vi "TEST FGV User Event Reference Manager.vi"(8 "error in (no error)":errorcluster) -> (0 "error out":errorcluster)   [LabVIEW 2011]
doc: "This is the solution for one of a two VI test process for the FGV User Event Reference.vi. This VI allows the operator to create an undertermined number of User Events and fire those User Events.\n\nAAL 9/09"
uses:
  Type Defs/TYPE FGV User Event Method.ctl
  Shared/QDMH Poly VIs/QDMH POLY Enqueue String.vi
panel:
  in  "Queue Name":string
  in  "Fire User Event":bool
  in  "User Event Ref to Act Upon":u16(ring)
  in  "Delete User Event":bool
  in  "Add User Event":bool
  out "Message Display":string
  in  "Cancel":bool
  in  "OK":bool
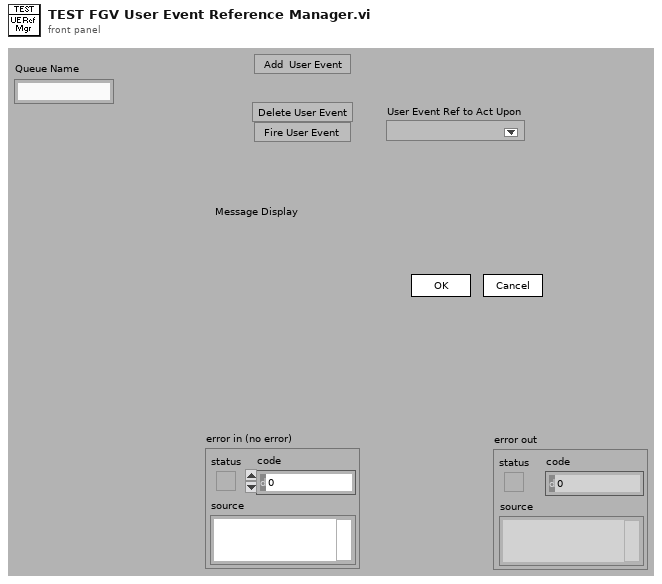
[diagram p1: front panel]
types:
  T1 = cluster{"Operator Name":string, "Current VI's Path":path, "# User Event  Refs":i32, "User Event #":i32, "User Event Names":string[], "User Event to Act Upon":i32}
  T2 = typedef "TYPE FGV User Event Method.ctl" = enum16{"Add User Event Ref", "Get User Event Ref", "Delete User Event Ref", "Get All User Event Refs", "Delete All User Event Refs"}
  T3 = typedef "TYPE FGV User Event Ref.ctl" = refnum<user-event>
  T4 = cluster{"User Event Name":string, "Variant":variant}
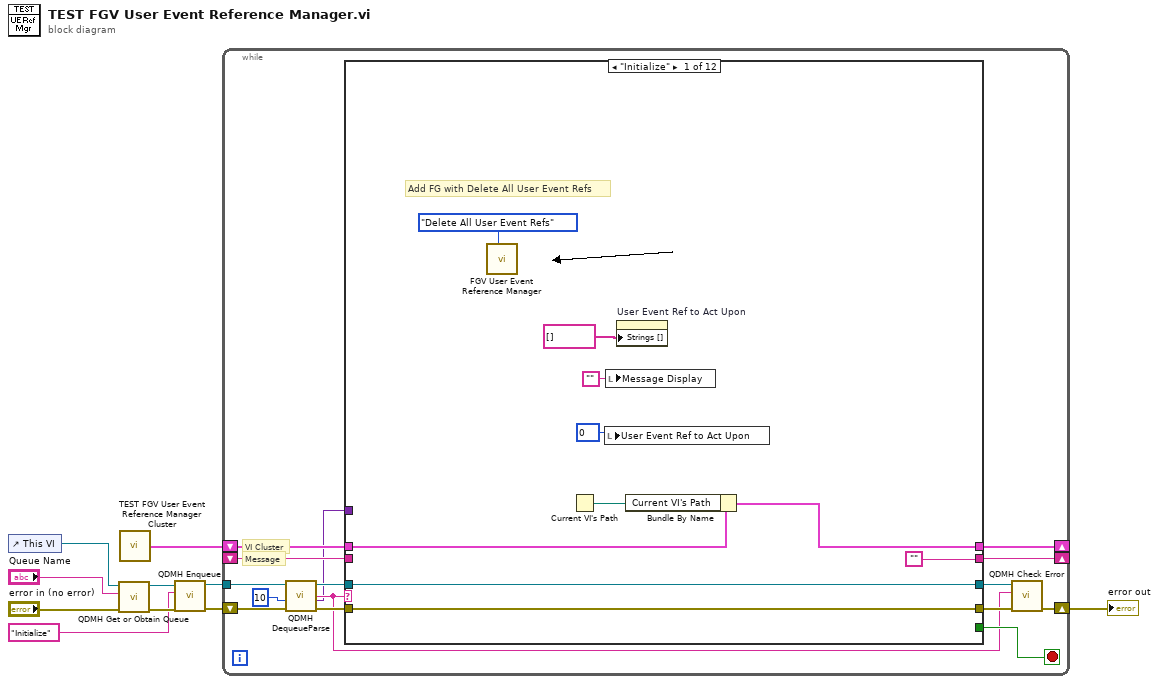
[diagram p0: block diagram]
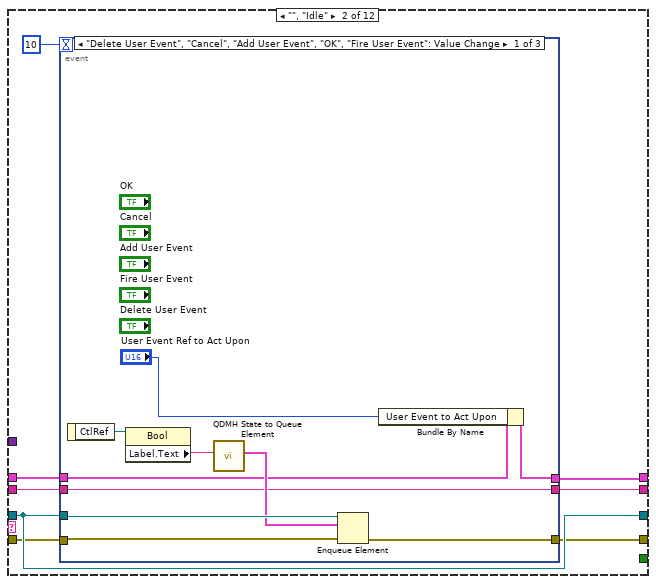
[diagram p2: hidden frame]
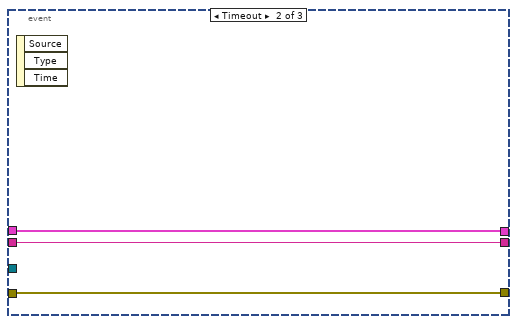
[diagram p3: hidden frame]
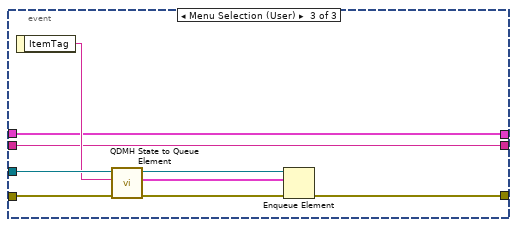
[diagram p4: hidden frame]
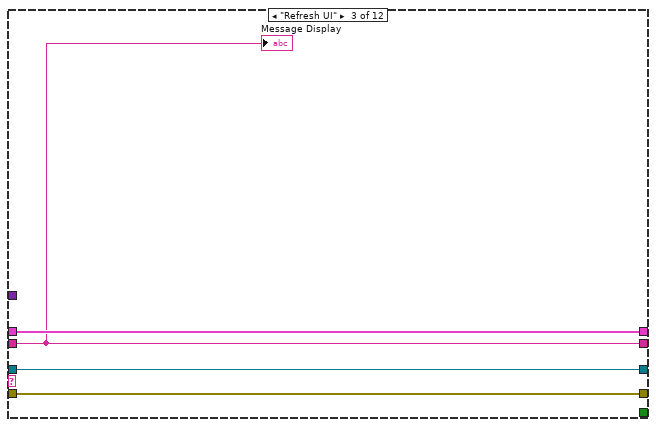
[diagram p5: hidden frame]
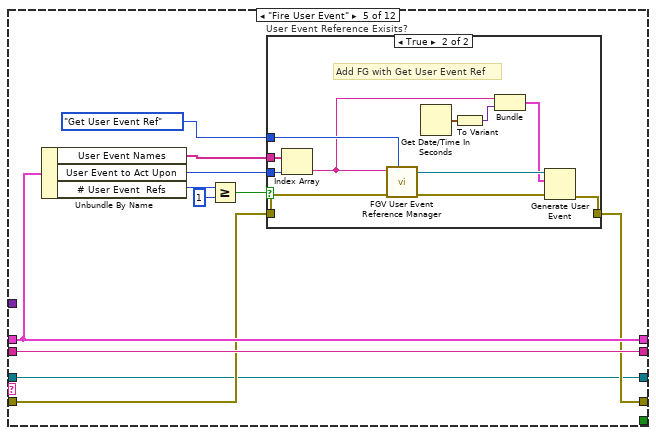
[diagram p7: hidden frame]
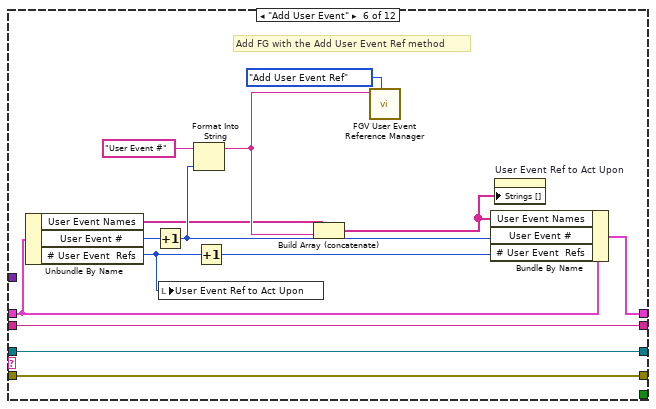
[diagram p9: hidden frame]
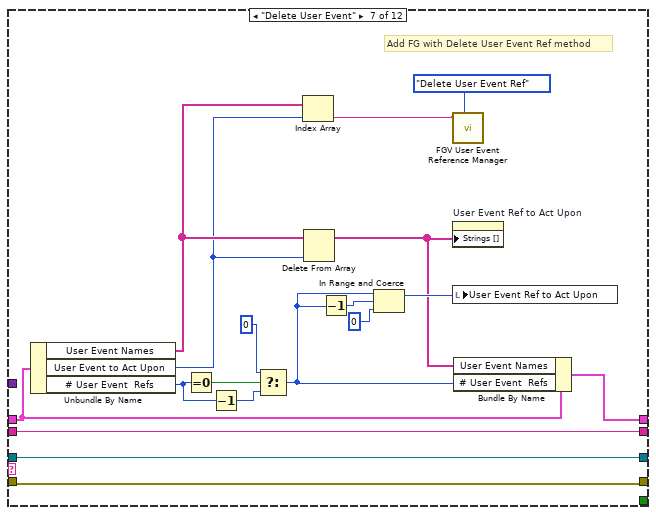
[diagram p10: hidden frame]
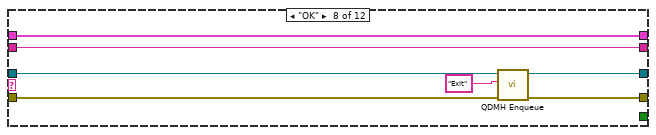
[diagram p11: hidden frame]
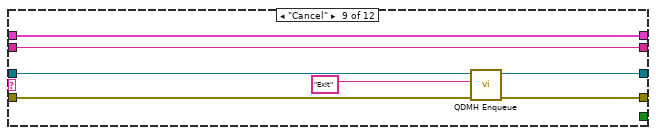
[diagram p12: hidden frame]
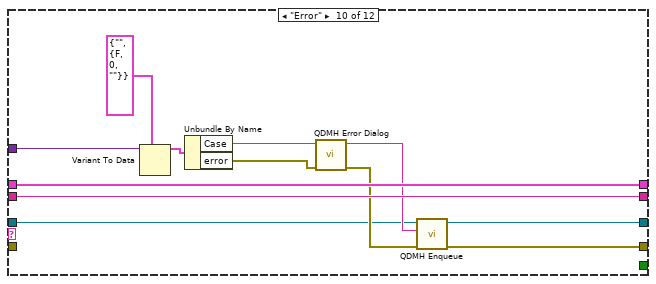
[diagram p13: hidden frame]
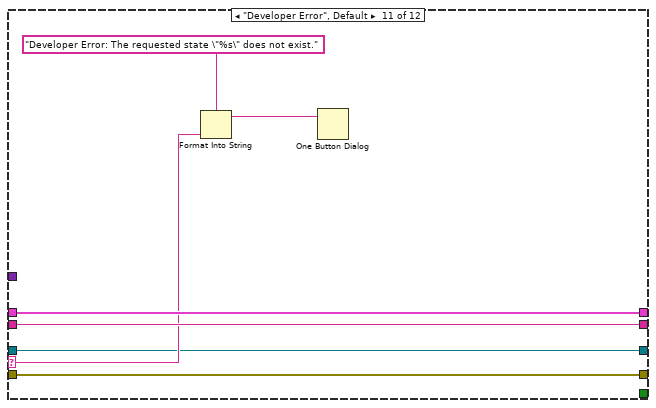
[diagram p14: hidden frame]
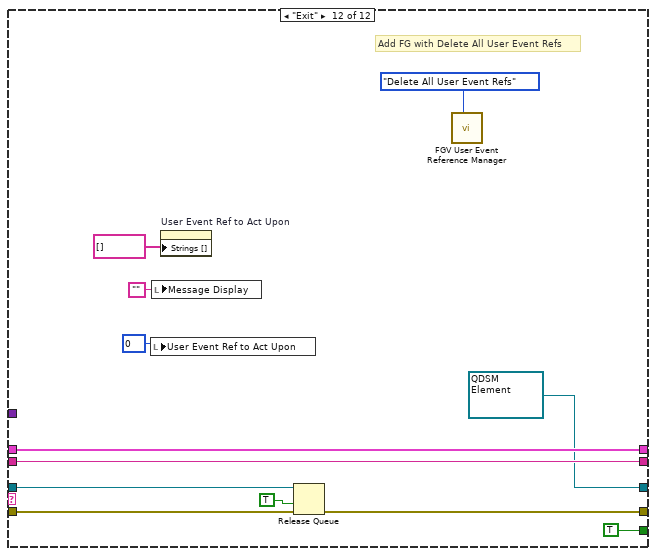
[diagram p15: hidden frame]
diagram:
  n1 = control-ref of="This VI"() -> (w2:refnum<vi>)
  n2 = call "QDMH Get or Obtain Queue.vi"("error in (no error)"="error in (no error)", "Queue Name"="Queue Name", "VI Refnum"=w2) -> ("error out"=w6:errorcluster, "queue out"=w9:refnum<queue>)  [unwired: 7 out]
  n3 = call "TEST FGV User Event Reference Manager Cluster.vi"() -> ("Cluster"=w8:T1)
  n4 = call-poly "QDMH Enqueue.vi"("error in (no error)"=w6, "State"="Initialize" ("element"), "queue"=w9) -> ("error out"=w7:errorcluster, "queue out"=w10:refnum<queue>)  [unwired: 7 out]
  n5 = while {
    tunnel: w10 -> [w21]
    shift-left: w8 -> [w22]
    shift-right: [w23] -> _
    shift-left: _ -> [w24]
    shift-right: [w15] -> _
    shift-right: [w13] -> w4
    shift-left: w7 -> [w17]
    stop <- w25 stop-if-true
    # "VI Cluster"
    # "Message"
    n6 = call "QDMH DequeueParse.vi"("error in (no error)"=w17, "Timeout"=10 ("ms timeout (-1)"), "queue"=w21) -> ("error out"=w18:errorcluster, "Variant Data"=w11:variant, "State"=w12:string, "queue out"=w19:refnum<queue>)  [unwired: 5 out]
    n7 = case shown="\"Initialize\"" w12 {
      selector: w12 -> [_ _ _ _ _ _ _ _ _ _ w156 _]
      tunnel: w19 -> [w26 w43 w64 w68 w72 w95 w109 w133 w140 w142 w153 w161]
      tunnel: [_ _ _ _ _ _ _ _ _ _ _ TRUE] -> w25
      tunnel: ["" w37 w66 w71 w82 w108 w126 w132 w139 w152 w159 w170] -> w15
      tunnel: w24 -> [_ w38 w66 w71 w82 w108 w126 w132 w139 w152 w159 w170]
      tunnel: [w33 w36 w67 w70 w81 w105 w124 w131 w138 w151 w158 w169] -> w23
      tunnel: w22 -> [w34 w39 w67 w70 w81 w106 w125 w131 w138 w151 w158 w169]
      tunnel: w18 -> [w35 w42 w65 w69 w77 w96 w111 w130 w137 _ w155 w167]
      tunnel: [w35 w41 w65 w69 w76 w96 w111 w129 w136 w143 w155 w166] -> w16
      tunnel: [w26 w43 w64 w68 w72 w95 w109 w127 w134 w144 w153 refnum<queue> refnum ("queue out")] -> w14
      tunnel: w11 -> [_ _ _ _ _ _ _ _ _ w141 _ _]
      frame "Initialize" {
        w28 = u16 0 items=[""] ("Queue to Delete")
        # "Add FG with Delete All User Event Refs"
        n8 = call "FGV User Event Reference Manager.vi"("Method (Get User Event Ref)"=TYPE_FGV_User_Event_Method."Delete All User Event Refs") -> ()  [unwired: 2 in, 9 out]
        n9 = Current VI's Path() -> (path=w32:path)
        n10 = local write "User Event Ref to Act Upon"(w28) -> ()
        n11 = local write "Message Display"("") -> ()
        n12 = property on="User Event Ref to Act Upon" class="Ring (strict)"("Strings []"=string[] []) -> ()  [unwired: 2 in, 2 out]
        n13 = Bundle By Name(cluster=w34, "Current VI's Path"=w32) -> (w33:T1)
      }
      frame "", "Idle" {
        n14 = event shown="[0] \"Delete User Event\", \"Cancel\", \"Add User Event\", \"OK\", \"Fire User Event\": Value Change" {
          selector: _ -> [_ _ _]
          dyn-events: _ -> [_ _ _]
          timeout: 10 -> [_ _ _]
          tunnel: w43 -> [w52 _ w63]
          tunnel: [w51 w56 w61] -> w41
          tunnel: w42 -> [w50 w56 w62]
          tunnel: w39 -> [w46 w55 w58]
          tunnel: w38 -> [w47 w54 w57]
          tunnel: [w45 w55 w58] -> w36
          tunnel: [w47 w54 w57] -> w37
          event "Delete User Event", "Cancel", "Add User Event", "OK", "Fire User Event": Value Change {
            n15 = event-data() -> ("CtlRef"=w53:refnum<vi>)  [unwired: 1 out]
            n16 = property class="Bool"(reference=w53) -> ("Label.Text"=w49:string)  [unwired: 1 in, 2 out]
            n17 = call "QDMH State to Queue Element.vi"("State"=w49) -> ("QDSM Element"=w48:cluster{"State":string, "Variant Data":variant})  [unwired: 10 out]
            n18 = Enqueue Element(queue=w52, element=w48, error in (no error)=w50) -> (error out=w51:errorcluster)  [unwired: 3 out]
            n19 = Bundle By Name(cluster=w46, "User Event to Act Upon"="User Event Ref to Act Upon") -> (w45:T1)
          }
          event Timeout {
            n20 = event-data() -> ()  [unwired: 4 out]
          }
          event Menu Selection (User) {
            n21 = event-data() -> ("ItemTag"=w60:string)  [unwired: 1 out]
            n22 = call "QDMH State to Queue Element.vi"("State"=w60) -> ("QDSM Element"=w59:cluster{"State":string, "Variant Data":variant})  [unwired: 10 out]
            n23 = Enqueue Element(queue=w63, element=w59, error in (no error)=w62) -> (error out=w61:errorcluster)  [unwired: 3 out]
          }
        }
      }
      frame "Refresh UI" {
        "Message Display" <- w66
      }
      frame "<add states as needed>" {
      }
      frame "Fire User Event" {
        n24 = Unbundle By Name(w81) -> ("User Event Names"=w80:string[], "User Event to Act Upon"=w78:i32, "# User Event  Refs"=w75:i32)
        n25 = Greater Or Equal?(x=w75, y=1) -> (x >= y?=w73:bool)
        n26 = case "User Event Reference Exisits?" shown="True" w73 {
          tunnel: w80 -> [_ w94]
          tunnel: TYPE_FGV_User_Event_Method."Get User Event Ref" ("Method (Get User Event Ref)") -> [_ w93]
          tunnel: w78 -> [_ w87]
          tunnel: w77 -> [w83 w85]
          tunnel: [w83 w84] -> w76
          frame False {
          }
          frame True {
            # "Add FG with Get User Event Ref"
            n27 = Index Array(array=w94, index=w87) -> (element=w92:string)
            n28 = call "FGV User Event Reference Manager.vi"("Method (Get User Event Ref)"=w93, "error in (no error)"=w85, "User Event Name"=w92) -> ("error out"=w86:errorcluster, "User Event Ref  Out"=w90:T3)  [unwired: 7 out]
            n29 = Get Date/Time In Seconds() -> (seconds since 1Jan1904=w91:timestamp)
            n30 = To Variant(anything=w91) -> (Variant=w89:variant)
            n31 = Bundle("User Event Name"=w92, "Variant"=w89) -> (w88:T4)  [unwired: 1 out]
            n32 = Generate User Event(user event=w90, event data cluster=w88, error in=w86) -> (error out=w84:errorcluster)  [unwired: 1 out]
          }
        }
      }
      frame "Add User Event" {
        # "Add FG with the Add User Event Ref method"
        n33 = Unbundle By Name(w106) -> ("User Event Names"=w99:string[], "User Event #"=w104:i32, "# User Event  Refs"=w97:i32)
        n34 = Increment(x=w104) -> (x+1=w103:i32)
        n35 = local write "User Event Ref to Act Upon"(w97) -> ()
        n36 = Format Into String(initial string="User Event #", w103) -> (resulting string=w100:string)  [unwired: 2 in, 1 out]
        n37 = Increment(x=w97) -> (x+1=w102:i32)
        n38 = Build Array (concatenate)(w99, w100) -> (w98:string[])
        n39 = call "FGV User Event Reference Manager.vi"("Method (Get User Event Ref)"=TYPE_FGV_User_Event_Method."Add User Event Ref", "User Event Name"=w100) -> ()  [unwired: 1 in, 9 out]
        n40 = Bundle By Name(cluster=w106, "User Event Names"=w98, "User Event #"=w103, "# User Event  Refs"=w102) -> (w105:T1)
        n41 = property on="User Event Ref to Act Upon" class="Ring (strict)"("Strings []"=w98) -> ()  [unwired: 2 in, 2 out]
      }
      frame "Delete User Event" {
        # "Add FG with Delete User Event Ref method"
        n42 = Unbundle By Name(w125) -> ("User Event Names"=w114:string[], "User Event to Act Upon"=w113:i32, "# User Event  Refs"=w122:i32)
        n43 = Equal To 0?(x=w122) -> (x = 0?=w123:bool)
        n44 = Decrement(x=w122) -> (x-1=w120:i32)
        n45 = Select(t=0 ("# Queue Refs"), s=w123, f=w120) -> (s? t:f=w117:i32)
        n46 = Index Array(array=w114, index=w113) -> (element=w115:string)
        n47 = Delete From Array(array=w114, index=w113) -> (array with subset deleted=w110:string[])  [unwired: 1 in, 1 out]
        n48 = Decrement(x=w117) -> (x-1=w119:i32)
        n49 = In Range and Coerce(upper limit=w117, x=w119, lower limit=0) -> (coerced(x)=w116:i32)  [unwired: 1 out]
        n50 = call "FGV User Event Reference Manager.vi"("Method (Get User Event Ref)"=TYPE_FGV_User_Event_Method."Delete User Event Ref", "User Event Name"=w115) -> ()  [unwired: 1 in, 9 out]
        n51 = property on="User Event Ref to Act Upon" class="Ring (strict)"("Strings []"=w110) -> ()  [unwired: 2 in, 2 out]
        n52 = local write "User Event Ref to Act Upon"(w116) -> ()
        n53 = Bundle By Name(cluster=w125, "User Event Names"=w110, "# User Event  Refs"=w117) -> (w124:T1)
      }
      frame "OK" {
        n54 = call-poly "QDMH Enqueue.vi"("error in (no error)"=w130, "State"="Exit" ("New State"), "queue"=w133) -> ("error out"=w129:errorcluster, "queue out"=w127:refnum<queue>)  [unwired: 7 out]
      }
      frame "Cancel" {
        n55 = call-poly "QDMH Enqueue.vi"("error in (no error)"=w137, "State"="Exit" ("New State"), "queue"=w140) -> ("error out"=w136:errorcluster, "queue out"=w134:refnum<queue>)  [unwired: 7 out]
      }
      frame "Error" {
        n56 = Variant To Data(type=cluster{"Case":string, "error":errorcluster} {"Case"="", "error"={"status"=FALSE, "code"=0, "source"=""}} ("QDSM Element"), Variant=w141) -> (data=w146:cluster{"Case":string, "error":errorcluster})  [unwired: 1 in, 1 out]
        n57 = Unbundle By Name(w146) -> ("Case"=w147:string, "error"=w148:errorcluster)
        n58 = call "QDMH Error Dialog.vi"("error"=w148, "Case Error Occured"=w147) -> ("error out (no error)"=w150:errorcluster, "Case to Execute"=w149:string)  [unwired: 8 out]
        n59 = call-poly "QDMH Enqueue.vi"("error in (no error)"=w150, "State"=w149, "queue"=w142) -> ("error out"=w143:errorcluster, "queue out"=w144:refnum<queue>)  [unwired: 7 out]
      }
      frame "Developer Error", Default {
        n60 = Format Into String(format string="Developer Error: The requested state \"%s\" does not exist." ("message"), w156) -> (resulting string=w154:string)  [unwired: 2 in, 1 out]
        n61 = One Button Dialog(message=w154) -> ()  [unwired: 2 out]
      }
      frame "Exit" {
        w163 = u16 0 items=[""] ("Queue to Delete")
        # "Add FG with Delete All User Event Refs"
        n62 = local write "User Event Ref to Act Upon"(w163) -> ()
        n63 = local write "Message Display"("") -> ()
        n64 = property on="User Event Ref to Act Upon" class="Ring (strict)"("Strings []"=string[] []) -> ()  [unwired: 2 in, 2 out]
        n65 = Release Queue(queue=w161, force destroy? (F)=TRUE, error in (no error)=w167) -> (error out=w166:errorcluster)  [unwired: 2 out]
        n66 = call "FGV User Event Reference Manager.vi"("Method (Get User Event Ref)"=TYPE_FGV_User_Event_Method."Delete All User Event Refs") -> ()  [unwired: 2 in, 9 out]
      }
    }
    n67 = call "QDMH Check Error.vi"("error in (no error)"=w16, "Case"=w12, "queue"=w14) -> ("error out"=w13:errorcluster)  [unwired: 1 in, 7 out]
  }
  "error out" <- w4
